vi "CDMA_TxCalDataNum.vi"(7 "ch_sf_tx":dbl, 8 "error in (no error)":errorcluster caption="错误输入（无错误）", 9 "coder_type":dbl, 10 "crc_num":dbl, 11 "Path":path) -> (0 "error out":errorcluster caption="错误输出", 1 "ch_cap":dbl, 2 "ch_bit_len":dbl, 3 "Path Out":path)   [LabVIEW 2015]
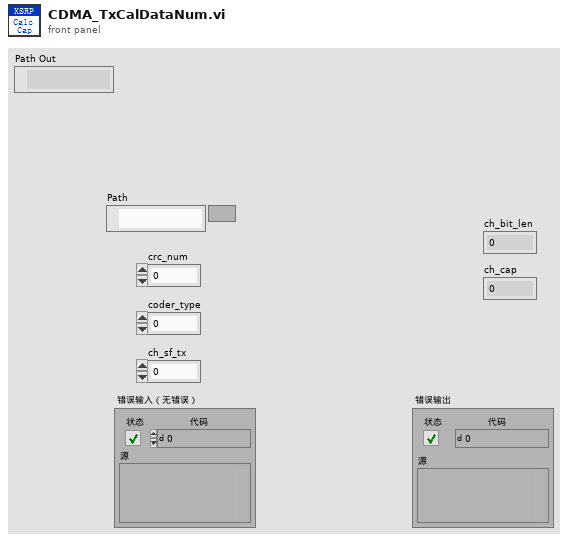
[diagram p1: front panel]
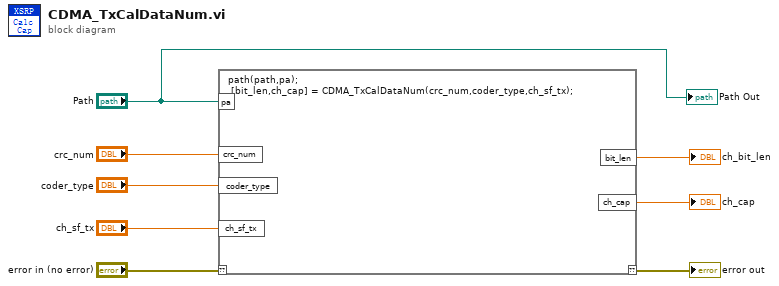
[diagram p0: block diagram]
diagram:
  n1 = script code="path(path,pa);\n [bit_len,ch_cap] = CDMA_TxCalDataNum(crc_num,coder_type,ch_sf_tx);"("??"="error in (no error)", "pa"="Path", "crc_num"="crc_num", "coder_type"="coder_type", "ch_sf_tx"="ch_sf_tx") -> ("??"=→"error out":errorcluster, "bit_len"=→"ch_bit_len":dbl, "ch_cap"=→"ch_cap":dbl)
  "Path Out" <- "Path"
